vi "SysLob Viewer Tabelle aufbereiten.vi"(7 "Cluster PC cRIO History File":T1, 8 "Fehler (in)":errorcluster caption="Fehlerkonstante", 9 "Cluster (in)":T2, 10 "Ebene":enum16{"PC+cRIO", "PC", "cRIO"}(ring), 11 "Table (Eingang)":refnum<vi>) -> (0 "Fehler (out)":errorcluster caption="Fehlerkonstante", 3 "Array-Typ (2D Dbl) out":string[][](array[string]))   [LabVIEW 2020, in "SysLog.lvlib"]
uses:
  SysLog.lvlib
  SysLogSort.ctl
  <vilib>/Utility/miscctls.llb/LVRowAndColumnTypeDef.ctl
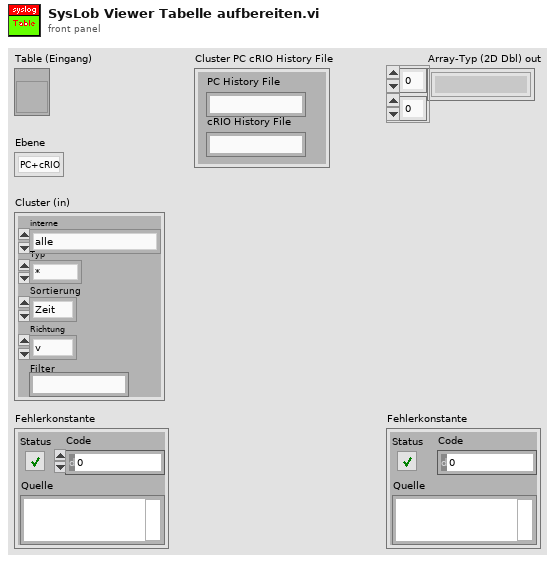
[diagram p1: front panel]
types:
  T1 = cluster{"PC History File":string, "cRIO History File":string}
  T2 = typedef "SysLog.lvlib/SysLogSort.ctl" = cluster{"interne":enum16{"alle", "nur benutzerrelevante", "nur interne"}, "Typ":enum16{"*", "Err+Warn", "Err", "Warn", "OK"}, "Sortierung":enum16{"Zeit", "Code", "Typ"}, "Richtung":enum16{"v", "^"}, "Filter":string}
  T3 = typedef "LVRowAndColumnTypeDef.ctl" = cluster{"Row":i32, "Column":i32}
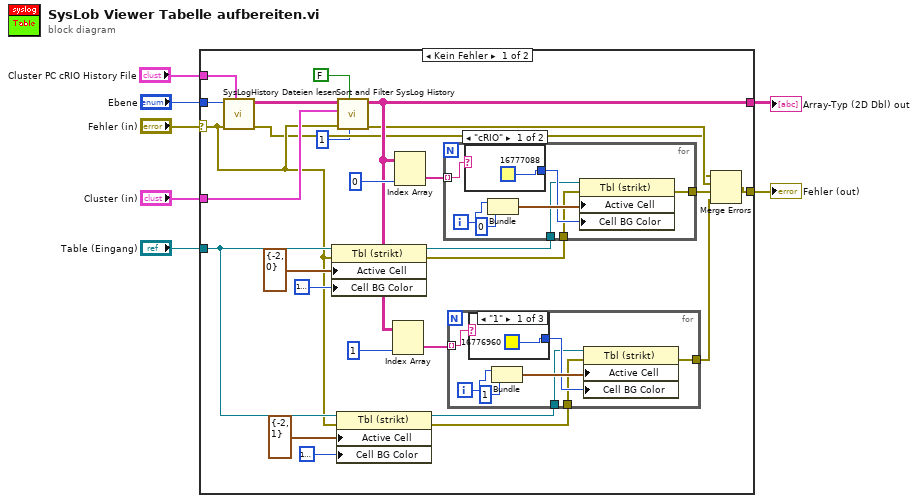
[diagram p0: block diagram]
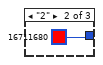
[diagram p2: hidden frame]
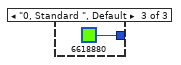
[diagram p3: hidden frame]
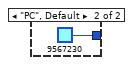
[diagram p4: hidden frame]
diagram:
  n1 = case shown="Kein Fehler" "Fehler (in)" {
    selector: "Fehler (in)" -> [w11 w55]
    tunnel: "Ebene" -> [w33 _]
    tunnel: "Cluster (in)" -> [w32 _]
    tunnel: [w19 _] -> w5
    tunnel: "Table (Eingang)" -> [w21 _]
    tunnel: [w15 w55] -> w3
    tunnel: "Cluster PC cRIO History File" -> [w13 _]
    frame No Error {
      n2 = call "SysLogHistory Dateien lesen.vi"("Cluster PC cRIO History File"=w13, "Fehler (in)"=w11, "Ebene"=w33) -> ("Fehler (out)"=w10:errorcluster, "Array-Typ (2D Dbl)"=w31:string[][])  [unwired: 7 in]
      n3 = property on="Eigenschaftsknoten" class="Tbl (strikt)"(reference=w21, error in=w11, "Active Cell"=T3 {"Row"=-2, "Column"=0} ("Aktive Zelle:Aktive Zelle"), "Cell BG Color"=u32 16777225) -> (reference out=w26:refnum<vi>, error out=w25:errorcluster)
      n4 = property on="Eigenschaftsknoten" class="Tbl (strikt)"(reference=w21, error in=w11, "Active Cell"=T3 {"Row"=-2, "Column"=1} ("Aktive Zelle:Aktive Zelle"), "Cell BG Color"=u32 16777225) -> (reference out=w17:refnum<vi>, error out=w16:errorcluster)
      n5 = call "Sort and Filter SysLog History.vi"("Spaltenindex intern"=u32 1, "NoSort"=FALSE, "Fehler (in)"=w11, "Cluster (in)"=w32, "Array-Typ (2D Dbl) in"=w31) -> ("Fehler (out)"=w12:errorcluster, "Array-Typ (2D Dbl) out"=w19:string[][])  [unwired: 5 in]
      n6 = Index Array(array=w19, index (col)=1 ("Deaktivierter Index (Spalte)")) -> (element=w18:string[])  [unwired: 1 in]
      n7 = Index Array(array=w19, index (col)=0 ("Deaktivierter Index (Spalte)")) -> (element=w30:string[])  [unwired: 1 in]
      n8 = for {
        tunnel: w30 -> [w50] mode=indexing
        tunnel: w26 -> [w47]
        tunnel: w25 -> [w46]
        tunnel: [w45] -> w28
        i -> [w51]
        n9 = case shown="\"cRIO\"" w50 {
          tunnel: [u32 16777088 u32 9567230] -> w48
          frame "cRIO" {
          }
          frame "PC", Default {
          }
        }
        n10 = Bundle(w51, "Deaktivierter Index (Spalte)"=0) -> (w49:cluster{i32, "Deaktivierter Index (Spalte)":i32})  [unwired: 1 in]
        n11 = property on="Eigenschaftsknoten" class="Tbl (strikt)"(reference=w47, error in=w46, "Active Cell"=w49, "Cell BG Color"=w48) -> (error out=w45:errorcluster)  [unwired: 1 out]
      }
      n12 = for {
        tunnel: w18 -> [w39] mode=indexing
        tunnel: w17 -> [w36]
        tunnel: w16 -> [w35]
        tunnel: [w34] -> w14
        i -> [w40]
        n13 = case shown="\"1\"" w39 {
          tunnel: [u32 16776960 u32 16711680 u32 6618880] -> w37
          frame "1" {
          }
          frame "2" {
          }
          frame "0, Standard ", Default {
          }
        }
        n14 = Bundle(w40, "Deaktivierter Index (Spalte)"=1) -> (w38:cluster{i32, "Deaktivierter Index (Spalte)":i32})  [unwired: 1 in]
        n15 = property on="Eigenschaftsknoten" class="Tbl (strikt)"(reference=w36, error in=w35, "Active Cell"=w38, "Cell BG Color"=w37) -> (error out=w34:errorcluster)  [unwired: 1 out]
      }
      n16 = Merge Errors(w10, w12, w28, w14) -> (w15:errorcluster)
    }
    frame Error {
    }
  }
  "Array-Typ (2D Dbl) out" <- w5
  "Fehler (out)" <- w3
